vi "数据提取.vi"(0 "输入缓冲":string, 1 "结束码":string="boot_end\r\n", 2 "数据大小":i32) -> (3 "数据大小判断":bool, 4 "数据完整性判断":bool, 5 "目标数据":string, 6 "剩余输出":string)   [LabVIEW 2017]
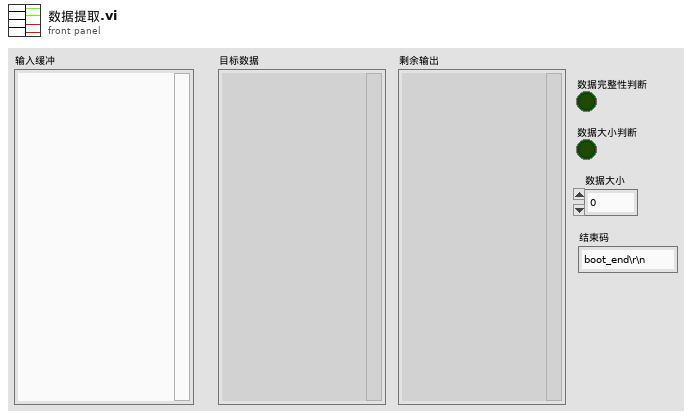
[diagram p1: front panel]
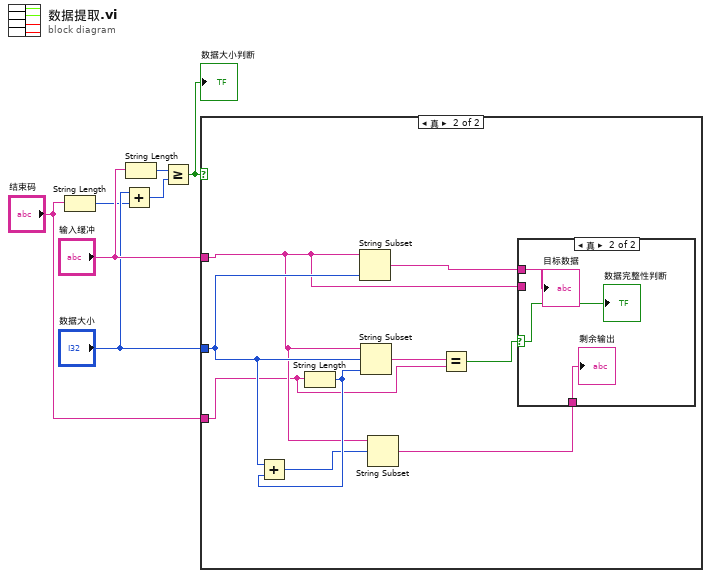
[diagram p0: block diagram]
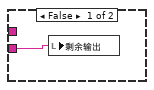
[diagram p3: hidden frame]
diagram:
  n1 = String Length(string="结束码") -> (length=w5:i32)
  n2 = Add(x="数据大小", y=w5) -> (x+y=w3:i32)
  n3 = String Length(string="输入缓冲") -> (length=w4:i32)
  n4 = Greater Or Equal?(x=w4, y=w3) -> (x >= y?=w2:bool)
  "数据大小判断" <- w2
  n5 = case shown="真" w2 {
    tunnel: "输入缓冲" -> [_ w9]
    tunnel: "数据大小" -> [_ w15]
    tunnel: "结束码" -> [_ w8]
    frame False {
    }
    frame True {
      n6 = String Length(string=w8) -> (length=w14:i32)
      n7 = Add(x=w15, y=w14) -> (x+y=w13:i32)
      n8 = String Subset(string=w9, length (rest)=w15) -> (substring=w16:string)  [unwired: 1 in]
      n9 = String Subset(string=w9, offset (0)=w15, length (rest)=w14) -> (substring=w11:string)
      n10 = String Subset(string=w9, offset (0)=w13) -> (substring=w12:string)  [unwired: 1 in]
      n11 = Equal?(x=w11, y=w8) -> (x = y?=w10:bool)
      n12 = case shown="真" w10 {
        selector: w10 -> [_ w18]
        tunnel: w16 -> [_ w20]
        tunnel: w12 -> [_ w19]
        tunnel: w9 -> [w17 _]
        frame False {
          n13 = local write "剩余输出"(w17) -> ()
        }
        frame True {
          "目标数据" <- w20
          "剩余输出" <- w19
          "数据完整性判断" <- w18
        }
      }
    }
  }
